vi "Clear_Charts.vi"(8 "error in (no error)":errorcluster, 11 "MHL_Data In":T1) -> (0 "error out":errorcluster, 3 "MHL_Data Out":T1)   [LabVIEW 2019, in "MHL.lvlib"]
uses:
  MHL.lvlib
  typedef/MHL_Data.ctl
  Alarm_Panel/Channel_Temperature_Threshold.ctl
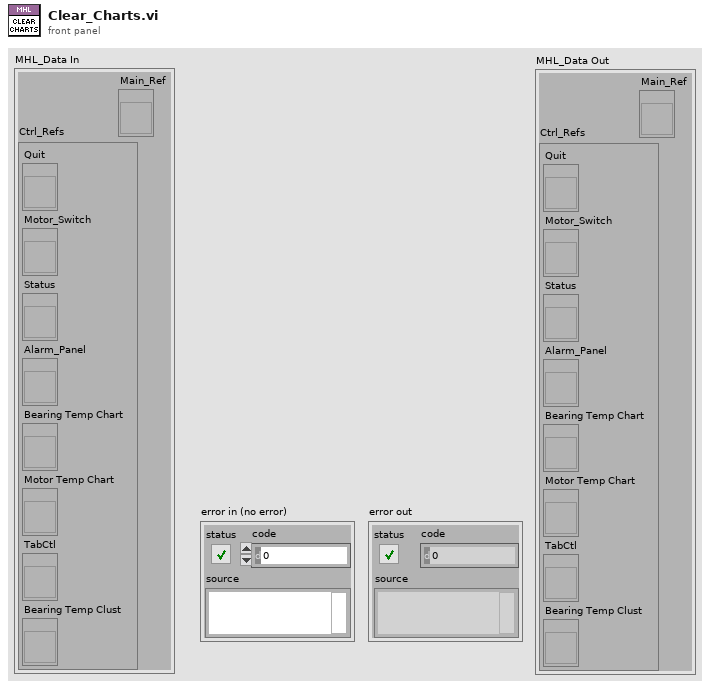
[diagram p1: front panel]
types:
  T1 = typedef "MHL.lvlib/MHL_Data.ctl" = cluster{"Ctrl_Refs":cluster{"Quit":refnum<vi>, "Motor_Switch":refnum<vi>, "Status":refnum<vi>, "Alarm_Panel":refnum<vi>, "Bearing Temp Chart":refnum<vi>, "Motor Temp Chart":refnum<vi>, "TabCtl":refnum<vi>, "Bearing Temp Clust":refnum<vi>}, "Main_Ref":refnum<vi>}
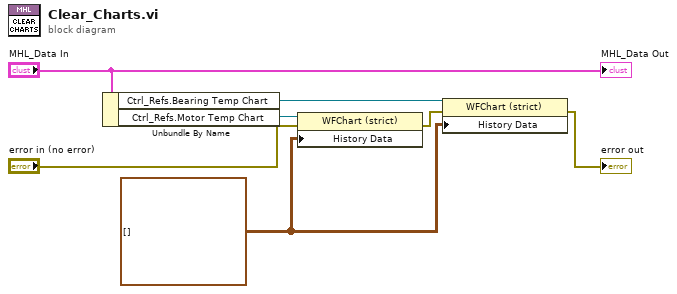
[diagram p0: block diagram]
diagram:
  w1 = waveform(dbl)[][] [] ("History Data")
  n1 = Unbundle By Name("MHL_Data In") -> ("Ctrl_Refs.Bearing Temp Chart"=w3:refnum<vi>, "Ctrl_Refs.Motor Temp Chart"=w6:refnum<vi>)
  n2 = property class="WFChart (strict)"(reference=w6, error in="error in (no error)", "History Data"=w1) -> (error out=w4:errorcluster)  [unwired: 1 out]
  n3 = property class="WFChart (strict)"(reference=w3, error in=w4, "History Data"=w1) -> (error out=→"error out":errorcluster)  [unwired: 1 out]
  "MHL_Data Out" <- "MHL_Data In"
